vi "Match Pattern part 3.vi"() -> ()   [LabVIEW 2020]
panel:
  out "after substring":string
  out "match substring":string
  out "before substring":string
  in  "string":string
  # "Part 3"
  # "Match Pattern"
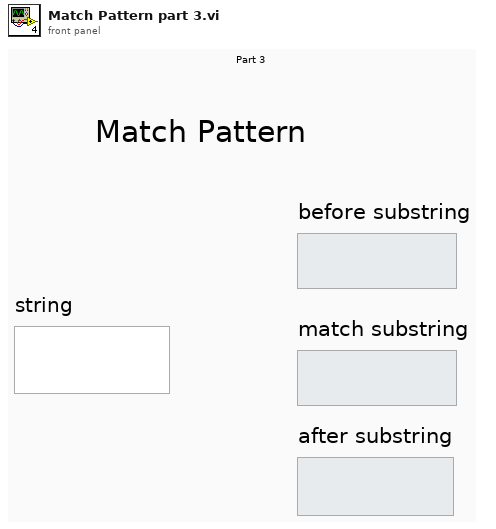
[diagram p1: front panel]
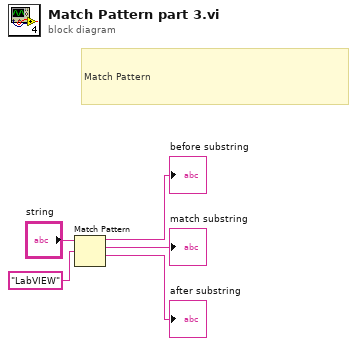
[diagram p0: block diagram]
diagram:
  # "Match Pattern"
  n1 = Match Pattern(string="string", regular expression="LabVIEW") -> (before substring=→"before substring":string, match substring=→"match substring":string, after substring=→"after substring":string)  [unwired: 1 in, 1 out]
